vi "new Bus Controller.vi"(8 "error in":errorcluster, 10 "BusController Config":T1={"scheduleMaxEntries"=512, "scheduleIDRef"=0, "triggerMode"=0, "eventLogOnHalt"=FALSE, "eventLogOnPause"=FALSE, "stepMode"=FALSE, "syncMode"=0, "defaultGap"=8.0, "timeout"=19.0} {"syncMode" items=["Selective", "All"]; "triggerMode" items=["None", "External", "Start"]}, 11 "name":string) -> (0 "error out":errorcluster, 3 "xml ref out":refnum<k24>)   [LabVIEW 2020, in "Ballard_1553_Hardware_ni.lvlib"]
uses:
  Ballard_1553_Hardware_ni.lvlib
  C:/Users/Administrator/Desktop/GIT/Ballard-MIL-STD-1553-Custom-Device/Source/System Explorer/SubVIs/Parse XML Ballard/1.2/BTIXML_SerDes.dll
  Ballard-MIL-STD-1553-Custom-Device/Source/System Explorer/SubVIs/Parse XML Ballard/1.2/BTIXML_SerDes.dll
  _typedefs/BusController_type.ctl
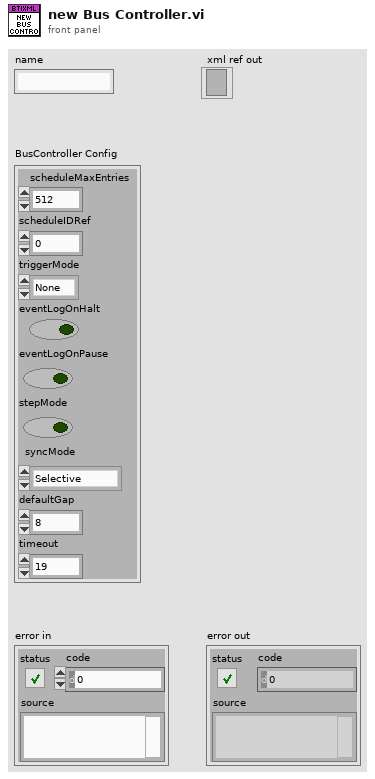
[diagram p1: front panel]
types:
  T1 = typedef "BusController_type.ctl" = cluster{"scheduleMaxEntries":u32, "scheduleIDRef":i32, "triggerMode":i32, "eventLogOnHalt":bool, "eventLogOnPause":bool, "stepMode":bool, "syncMode":i32, "defaultGap":dbl, "timeout":dbl}
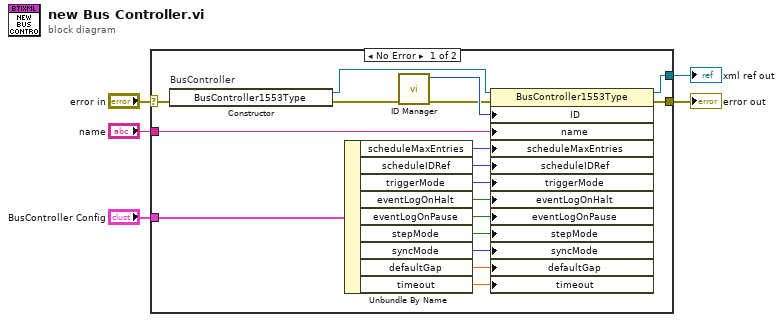
[diagram p0: block diagram]
diagram:
  n1 = case shown="No Error" "error in" {
    selector: "error in" -> [w23 w24]
    tunnel: [w22 w24] -> w4
    tunnel: [w21 _] -> w3
    tunnel: "BusController Config" -> [w19 _]
    tunnel: "name" -> [w6 _]
    frame No Error {
      n2 = constructor on="BusController" class="BusController1553Type"(error in=w23) -> (reference out=w20:refnum<k24>, error out=w9:errorcluster)  [unwired: 2 in, 1 out]
      n3 = Unbundle By Name(w19) -> ("scheduleMaxEntries"=w18:u32, "scheduleIDRef"=w17:i32, "triggerMode"=w16:i32, "eventLogOnHalt"=w15:bool, "eventLogOnPause"=w14:bool, "stepMode"=w13:bool, "syncMode"=w12:i32, "defaultGap"=w11:dbl, "timeout"=w10:dbl)
      n4 = call "ID Manager.vi"("error in"=w9) -> ("error out"=w7:errorcluster, "ID out"=w8:i32)  [unwired: 9 in]
      n5 = property class="BusController1553Type"(reference=w20, error in=w7, "ID"=w8, "name"=w6, "scheduleMaxEntries"=w18, "scheduleIDRef"=w17, "triggerMode"=w16, "eventLogOnHalt"=w15, "eventLogOnPause"=w14, "stepMode"=w13, "syncMode"=w12, "defaultGap"=w11, "timeout"=w10) -> (reference out=w21:refnum<k24>, error out=w22:errorcluster)
    }
    frame Error {
    }
  }
  "error out" <- w4
  "xml ref out" <- w3
